vi "calculateSearchDirectories.vi"(11 "TestStand 1 course folder name":string="Developing Test Programs") -> (2 "Search Directories to Remove":path[](array[path]), 3 "Search Directories to Add":path[](array[path]))   [LabVIEW 2013]
uses:
  <vilib>/registry/registry.llb/Registry RtKey.ctl
  <vilib>/registry/registry.llb/Registry View.ctl
  <vilib>/registry/registry.llb/Registry SAM.ctl
  <vilib>/registry/registry.llb/Read Registry Value Simple STR.vi
panel:
  out "error out":errorcluster
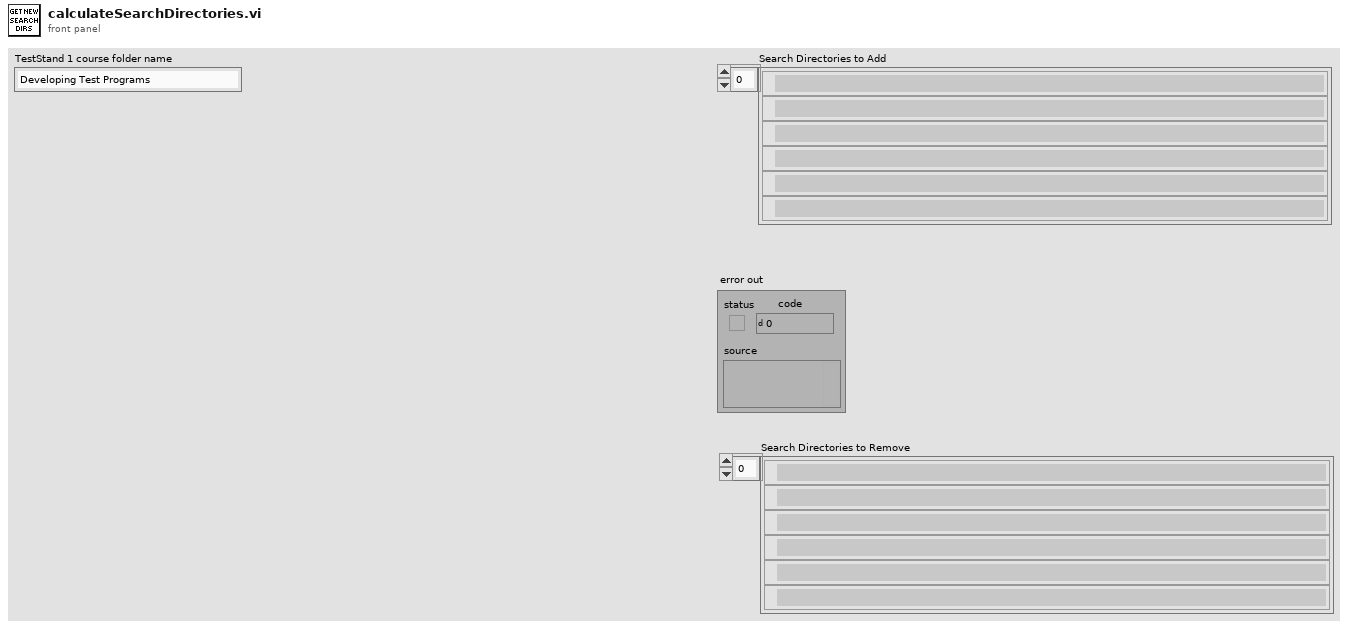
[diagram p1: front panel]
types:
  T1 = typedef "Registry SAM.ctl" = enum32{"KEY_QUERY_VALUE", "KEY_SET_VALUE", "KEY_CREATE_SUB_KEY", "KEY_ENUMERATE_SUB_KEYS", "KEY_NOTIFY", "KEY_CREATE_LINK", "KEY_READ", "KEY_WRITE", "KEY_ALL_ACCESS", "KEY_READ | KEY_WRITE"}
  T2 = typedef "Registry View.ctl" = u16
  T3 = typedef "Registry RtKey.ctl" = enum32{"HKEY_CLASSES_ROOT", "HKEY_CURRENT_USER", "HKEY_LOCAL_MACHINE", "HKEY_USERS", "HKEY_PERFORMANCE_DATA", "HKEY_CURRENT_CONFIG", "HKEY_DYN_DATA"}
  T4 = typedef "Registry refnum.ctl" = refnum<k1>
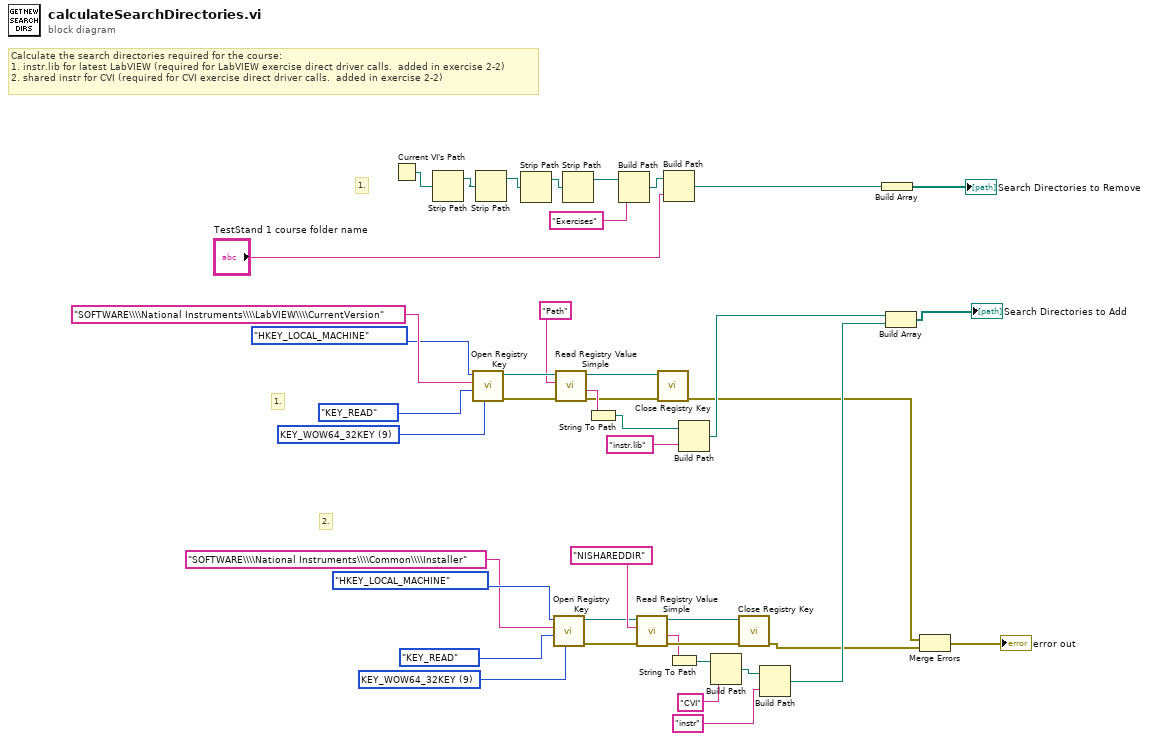
[diagram p0: block diagram]
diagram:
  w21 = T2 9 items=["Default"=0, "KEY_WOW64_64KEY"=8, "KEY_WOW64_32KEY"=9] ("registry view")
  w34 = T2 9 items=["Default"=0, "KEY_WOW64_64KEY"=8, "KEY_WOW64_32KEY"=9] ("registry view")
  # "1."
  # "2."
  # "1."
  # "Calculate the search directories required for the course:\n1. instr.lib for latest LabVIEW (required for LabVIEW exercise direct driver calls.  added in exercise 2-2)\n2. shared instr for CVI (required for CVI exercise direct driver calls.  added in exercise 2-2)"
  n1 = Current VI's Path() -> (path=w5:path)
  n2 = Strip Path(path=w5) -> (stripped path=w6:path)  [unwired: 1 out]
  n3 = call <vilib>:"Open Registry Key.vi"("registry view"=w21, "security access mask (KEY_READ | KEY_WRITE)"=Registry_SAM."KEY_READ", "subkey"="SOFTWARE\\\\National Instruments\\\\LabVIEW\\\\CurrentVersion", "root key (HKEY_LOCAL_MACHINE)"=Registry_RtKey."HKEY_LOCAL_MACHINE") -> ("error out"=w24:errorcluster, "refnum out"=w25:T4)  [unwired: 6 in]
  n4 = Strip Path(path=w6) -> (stripped path=w3:path)  [unwired: 1 out]
  n5 = Strip Path(path=w3) -> (stripped path=w7:path)  [unwired: 1 out]
  n6 = call <vilib>:"Open Registry Key.vi"("registry view"=w34, "security access mask (KEY_READ | KEY_WRITE)"=Registry_SAM."KEY_READ", "subkey"="SOFTWARE\\\\National Instruments\\\\Common\\\\Installer", "root key (HKEY_LOCAL_MACHINE)"=Registry_RtKey."HKEY_LOCAL_MACHINE") -> ("error out"=w31:errorcluster, "refnum out"=w30:T4)  [unwired: 6 in]
  n7 = call-poly <vilib>:"Read Registry Value Simple.vi"("error in (no error)"=w24, "value"="Path", "refnum"=w25) -> ("error out"=w18:errorcluster, "String/Binary data"=w19:string, "refnum out"=w17:T4)  [unwired: 3 in, 1 out]
  n8 = Strip Path(path=w7) -> (stripped path=w8:path)  [unwired: 1 out]
  n9 = String To Path(string=w19) -> (path=w15:path)
  n10 = Build Path(base path=w8, name or relative path="Exercises") -> (appended path=w9:path)
  n11 = call-poly <vilib>:"Read Registry Value Simple.vi"("error in (no error)"=w31, "value"="NISHAREDDIR", "refnum"=w30) -> ("error out"=w39:errorcluster, "String/Binary data"=w37:string, "refnum out"=w40:T4)  [unwired: 3 in, 1 out]
  n12 = call <vilib>:"Close Registry Key.vi"("error in (no error)"=w18, "refnum"=w17) -> ("error out"=w12:errorcluster)  [unwired: 5 in]
  n13 = Build Path(base path=w9, name or relative path="TestStand 1 course folder name") -> (appended path=w2:path)
  n14 = String To Path(string=w37) -> (path=w36:path)
  n15 = Build Path(base path=w15, name or relative path="instr.lib") -> (appended path=w14:path)
  n16 = Build Path(base path=w36, name or relative path="CVI") -> (appended path=w29:path)
  n17 = call <vilib>:"Close Registry Key.vi"("error in (no error)"=w39, "refnum"=w40) -> ("error out"=w13:errorcluster)  [unwired: 5 in]
  n18 = Build Path(base path=w29, name or relative path="instr") -> (appended path=w27:path)
  n19 = Build Array(w2) -> (→"Search Directories to Remove":path[])
  n20 = Build Array(w14, w27) -> (→"Search Directories to Add":path[])
  n21 = Merge Errors(w12, w13) -> (→"error out":errorcluster)
